vi "test_verify_search.vi"() -> ()   [LabVIEW 2015]
uses:
  _SubVIs/Advanced/search-double.vi
  binary_search.lvlib
panel:
  out "Error?":bool
  in  "Passes":i32=10000
  in  "Elements to Generate":i32=100000
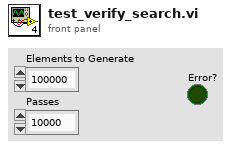
[diagram p1: front panel]
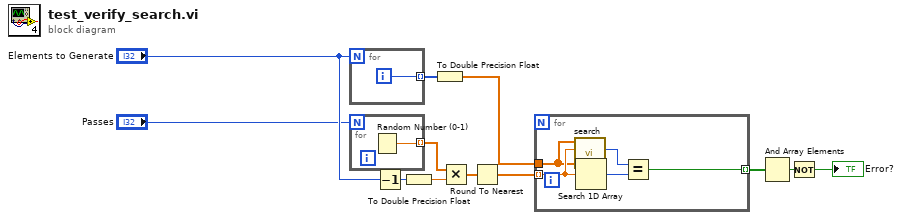
[diagram p0: block diagram]
diagram:
  n1 = for {
    N: "Elements to Generate" -> [_]
    tunnel: [w13] -> w7 mode=indexing
    i -> [w13]
  }
  n2 = for {
    N: "Passes" -> [_]
    tunnel: [w14] -> w6 mode=indexing
    n3 = Random Number (0-1)() -> (number: 0 to 1=w14:dbl)
  }
  n4 = Decrement(x="Elements to Generate") -> (x-1=w3:i32)
  n5 = To Double Precision Float(number=w3) -> (double precision float=w5:dbl)
  n6 = To Double Precision Float(number=w7) -> (double precision float=w8:dbl[])
  n7 = Multiply(x=w6, y=w5) -> (x*y=w4:dbl[])
  n8 = Round To Nearest(number=w4) -> (nearest integer value=w9:dbl[])
  n9 = for {
    tunnel: w8 -> [w15]
    tunnel: w9 -> [w19] mode=indexing
    tunnel: [w16] -> w2 mode=indexing
    n10 = call-poly "search.vi"("Search"=w19, "Data (dbl) []"=w15) -> ("Index"=w18:i32)  [unwired: 9 in]
    n11 = Search 1D Array(1D array=w15, element=w19) -> (index of element=w17:i32)  [unwired: 1 in]
    n12 = Equal?(x=w18, y=w17) -> (x = y?=w16:bool)
  }
  n13 = And Array Elements(Boolean array=w2) -> (logical AND=w12:bool)
  n14 = Not(x=w12) -> (.not. x?=→"Error?":bool)
